vi "Main FPGA 5-axis Servo 3.vi"() -> ()   [LabVIEW 2014]
uses:
  <vilib>/Motion/MotorControl/_s/nism.encoder.config.ctl
  <vilib>/Motion/MotorControl/_s/nism.encoder.incremental.config.ctl
  <vilib>/Motion/MotorControl/_s/nism.incremental.indexCriteria.ctl
  <vilib>/Motion/MotorControl/_s/nism.mdoMemoryOffsets.ctl
  <vilib>/Motion/MotorControl/_s/nism.pid.gains.fxp.18.ctl
  <vilib>/Motion/MotorControl/_s/nism.pi.v.outputRange.fxp.6.12.ctl
  <vilib>/Motion/MotorControl/_s/nism.interpretControlRegister.stateTransition.ctl
  <vilib>/Platform/TimedLoop/XDataNode/timing_clust.ctl
  <vilib>/Platform/TimedLoop/XDataNode/nitl_modes.ctl
  <vilib>/Platform/TimedLoop/XDataNode/wakeup.ctl
  <vilib>/Motion/MotorControl/_s/nism.digitalInputs.portA.ctl
  <vilib>/rvi/Emulation/niFpgaGetClockAttributes.vi
  <vilib>/rvi/Emulation/niFpgaSctlEmulationGetInTimedLoop.vi
  <vilib>/rvi/Emulation/niFpgaEmulationReportErrorSimple.vi
  Global FPGA 6-axis.vi
  <vilib>/Motion/MotorControl/_s/nism.interpretControlRegister.indexed.vi
  <vilib>/rvi/Emulation/niFpgaProcessEmulError.vi
  <vilib>/Motion/MotorControl/_s/nism.mdo.read.encoder.vi
  <vilib>/Motion/MotorControl/_s/nism.mdo.read.positionLoopSyncData.vi
  <vilib>/Motion/MotorControl/_s/nism.mdo.read.splineData.vi
  <vilib>/Motion/MotorControl/_s/nism.mdo.read.single.vi
  <vilib>/Motion/MotorControl/_s/nism.generateStatusRegister.indexed.vi
  <vilib>/rvi/eio/common/nirviEmuTemplateMethod_errors.vi
  <vilib>/rvi/Emulation/niFpgaCriticalErrorInLSC.vi
  <vilib>/Motion/MotorControl/_s/nism.splineInterpolation.fxp.3.index.vi
  <vilib>/Motion/MotorControl/_s/nism.pid.simple.fxp.index.2.vi
  <vilib>/Motion/MotorControl/_s/nism.mdo.handler.indexed.vi
  <vilib>/Motion/MotorControl/_s/nism.digitalFilter.indexed.vi
  <vilib>/Motion/MotorControl/_s/nism.interpretDIOControl.portA.multiple.vi
  <vilib>/Motion/MotorControl/_s/nism.generateDIOStatus.portA.indexed.2.vi
  <vilib>/Motion/SoftMotion/Synchronization/nism.rioScan.generateSyncScan.vi
  <vilib>/Motion/MotorControl/_s/nism.incremental.p.2.vi
  <vilib>/eio/EIONode/EIONode.xnode
  <vilib>/Platform/TimedLoop/XDataNode/XDataNode.xnode
  <vilib>/Motion/MotorControl/NI_SoftMotion_MotorControlIP.lvlib
  <vilib>/Platform/TimedLoop/XDataNode/XDNodeRunTimeDep.lvlib
  <vilib>/Motion/SoftMotion/Synchronization/NI_SoftMotion_Synchronization.lvlib
  <vilib>/rvi/Analysis/measure/butterworth/XNode/niFpgaButterworthFilter.xnode
panel:
  in  "Reset Encoder 2":bool caption="reset"
  out "Velocity Feedback":i16[](array[numeric])
  out "pos. error":i16[](array[numeric])
  out "pos. error exceeded":bool[](array[boolean])
  in  "calls per sample (vel)":u16=2000 caption="calls per sample"
  out "Axis States":T1[](array[typedef])=[enum."Invalid", enum."Invalid", enum."Invalid", enum."Invalid", enum."Invalid", enum."Invalid"]
  in  "Limit Ranges":T2[](array[typedef])=[{"output low"=0.0, "output high"=0.0}, {"output low"=0.0, "output high"=0.0}, {"output low"=0.0, "output high"=0.0}, {"output low"=0.0, "output high"=0.0}, {"output low"=0.0, "output high"=0.0}, {"output low"=0.0, "output high"=0.0}]
  in  "Gains":T3[](array[typedef])=[{"kp"=0.0, "kd"=0.0, "ki"=0.0}, {"kp"=0.0, "kd"=0.0, "ki"=0.0}, {"kp"=0.0, "kd"=0.0, "ki"=0.0}, {"kp"=0.0, "kd"=0.0, "ki"=0.0}, {"kp"=0.0, "kd"=0.0, "ki"=0.0}, {"kp"=0.0, "kd"=0.0, "ki"=0.0}]
  out "AO Check":fxp<+/-,20,5>[](array[numeric])
  in  "AO Manual":fxp<+/-,20,5>[](array[numeric])=[0.0, 0.0, 0.0, 0.0, 0.0, 0.0]
  out "Position Feedback":i32[](array[numeric])
  in  "Reset Encoder 1":bool caption="reset"
  out "corrected period":u16
  in  "AO Disabled?":bool
  out "PID loop time (ticks)":u32
  in  "AO Override?":bool
  in  "position error limit":i16=10000
  out "SE value":u32 caption="value"
  in  "Memory Type":T4=90 caption="mbox memory offsets" items=["1 / Current Loop Rate"=108, "Anti-Resonance Enable Velocity"=98, "Axis Control Mode"=88, "Axis Velocity Filter Coefficient 1"=60, "Axis Velocity Filter Coefficient 2"=61, "Axis Velocity Filter Coefficient 3"=62, "Axis Velocity Filter Frequency"=59, "Captured Index Position"=68, "Captured Position"=58, "Coefficient 0"=96, "Coefficient 1"=95, "Coefficient 2"=101, "Coefficient 3"=97, "Coefficient 4"=99, "Coefficient 5"=100, "Compare Mode"=81, "Compare Period"=32, "Compare Position"=55, "Config Sent"=82, "Control Register"=33, "Control Register State Transition"=57, "Current Loop I2T Constant"=38, "Current Loop I2T Current to Clamp to"=40, "Current Loop I2T Icont Limit Squared"=39, "Current Loop Integral Gain"=36, "Current Loop Proportional Gain"=35, "Current Loop Rate"=37, "Digital Input Digital Filter"=1, "Digital Output Safe State"=73, "Encoder Filter Rate (uS)"=92, "Encoder Index Active State"=65, "Encoder Index Reference Line A State"=66, "Encoder Index Reference Line B State"=67, "Encoder Line A Active State"=63, "Encoder Line B Active State"=64, "Encoder Velocity"=90, "Enforce Open-Loop Position Error Limit"=71, "Fault Codes"=45, "Fault Occurred"=41, "Forward Limit Digital Filter"=24, "Gain Set 2 Current Loop Integral Gain"=106, "Gain Set 2 Current Loop Proportional Gain"=107, "Home Switch Digital Filter"=26, "Maximum Position Error Exceeded"=69, "Motor Hall Angle 1"=12, "Motor Hall Angle 2"=13, "Motor Hall Angle 3"=14, "Motor Peak Current"=16, "Motor Peak Time"=17, "Motor Phase Current Offset(A)"=83, "Motor Phase Current Offset(B)"=84, "Motor Poles"=18, "Motor Rated Phase Current"=15, "Null"=0, "PWM Periods Per Tick"=94, "Position Capture Active State"=56, "Position Capture Condition"=30, "Position Capture Digital Filter"=31, "Position Compare Action"=27, "Position Compare Active State"=54, "Position Compare Pulse Width"=29, "Position Compare Safe State"=72, "Position Compare Window"=28, "Position Loop Period"=103, "Position Loop Position Error Limit"=70, "Position Loop Proportional Gain"=9, "Reverse Limit Digital Filter"=25, "Scan Period (nsec)"=104, "Spline Period/Trajectory Period"=44, "Spline Type"=42, "Status Register"=34, "Stepper Current Reduction Delay"=20, "Stepper Current Reduction Percentage"=19, "Stepper Microstepping Rate"=21, "Stepper Minimum Pulse Width"=22, "Stepper Reduced Current"=85, "Stepper Spline Loop Period"=23, "Torque Smoothing Gain"=102, "Torque Smoothing Phase"=105, "Trajectory Period/Spline Period"=43]
  in  "Encoder filter value (us) Manual":u16=10
  out "encoder config":T5
  in  "Velocity Filter Active?":bool
  in  "Encoder Config (Manual)":T5={"active states"={"line a active high?"=FALSE, "line b active high?"=FALSE, "index active high?"=FALSE}, "index criteria"={"a"=FALSE, "b"=FALSE, "z"=FALSE}, "vel. filter coeffs."=[0, 0, 0]} caption="encoder config"
  out "Home Limits":bool[](array[boolean])
  out "Fwd Limits":bool[](array[boolean])
  out "Rev Limits":bool[](array[boolean])
  out "Drive Enable":bool[](array[boolean])
  in  "Enable Watchdog":bool
  in  "Pet Watchdog":bool
  in  "Watchdog Timeout Period (ticks)":u64=40000000 format="%.0p"
  out "Watchdog Timed Out?":bool
  out "Time Since Last Pet":u64
  in  "Enable value":bool
  in  "Drive Enable override?":bool
  in  "Sync Value":bool
  in  "Sync Enable override?":bool
  in  "Invert direction?":bool
  out "Sync is Fault":bool
  out "Sync is Locked":bool
  # "Synchronization Loop"
  # "Control Status Loop"
  # "Notes: \n1. This VI provides the communication interface between the NI SoftMotion Engine and the LabVIEW FPGA Module. You must compile this VI for a specific FPGA target before use. After compiling, run the VI before running any of the Express VI examples. For information on moving this example to another FPGA target, refer to ni.com/info and enter info code fpgaex.\n\n2. Only use the Reset Axis button if you are unable to communicate with the axis by any other means. This button resets the device state machine and other VIs to a known state. After resetting the axis, switch the NI Scan Engine from Active Mode to Configuration Mode, then back to Active Mode, before attempting to enable the axis."
  # "(These two buttons \nare for testing\npurposes.)"
  # "(These two buttons \nare for testing\npurposes.)"
  # "Position/PID Loop"
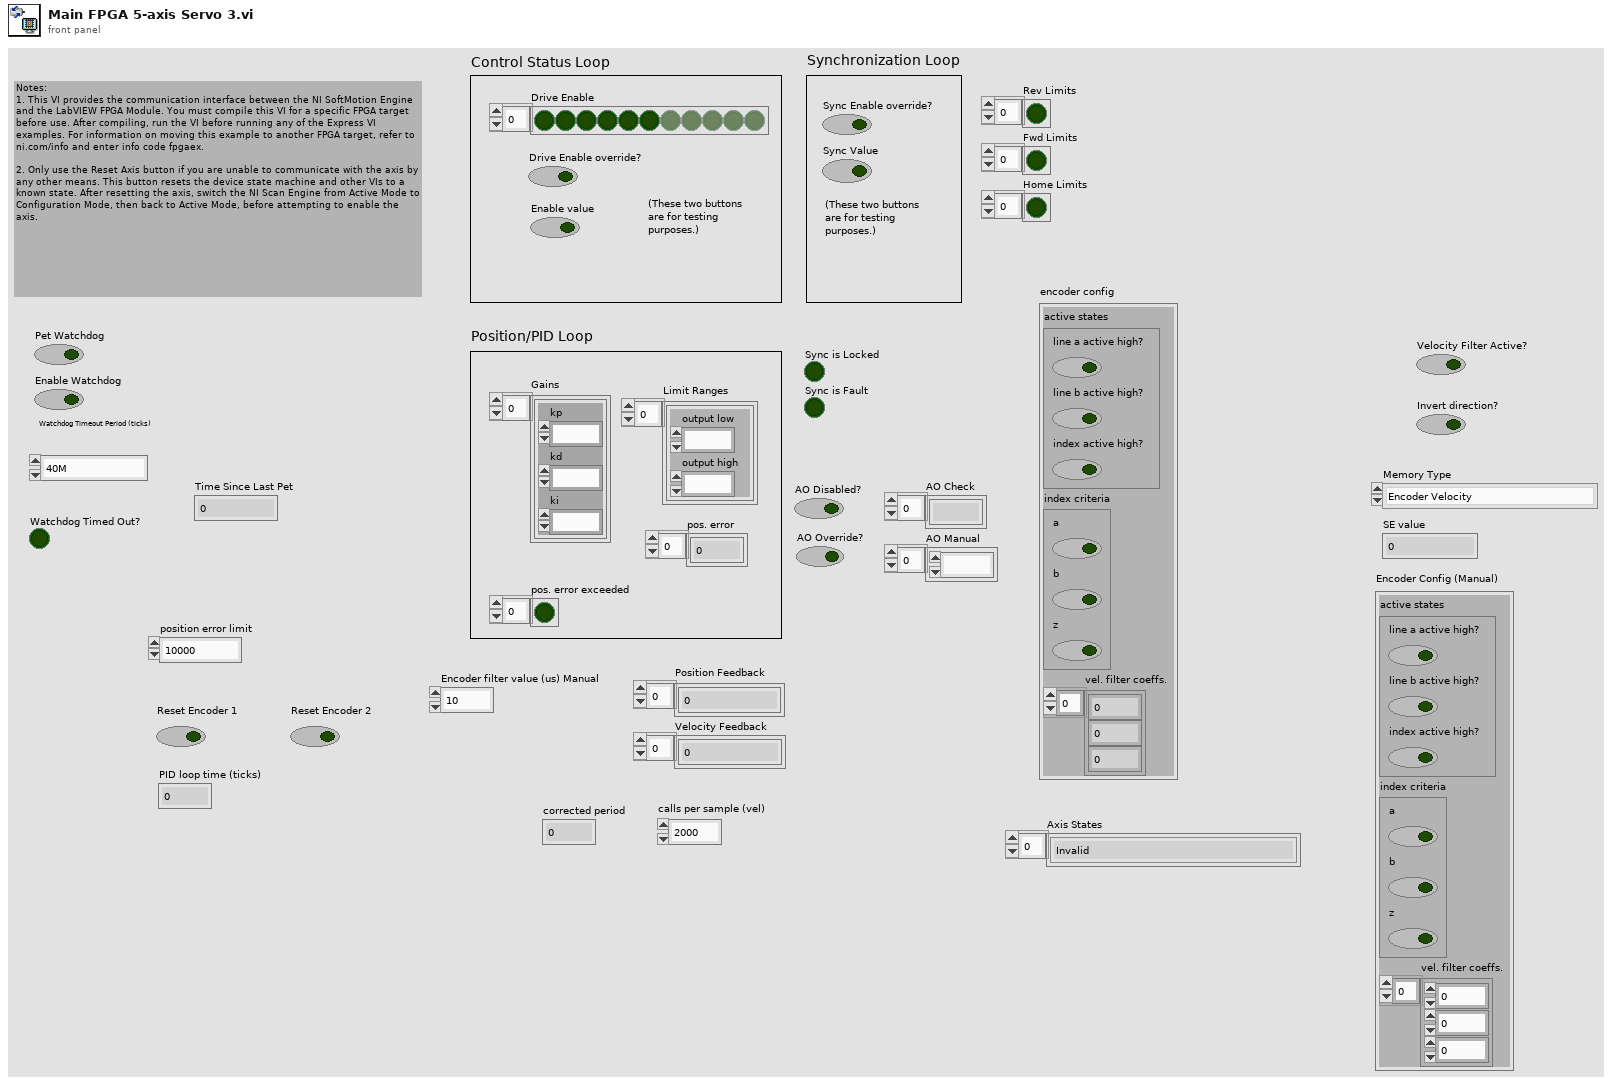
[diagram p1: front panel]
types:
  T1 = typedef "NI_SoftMotion_MotorControlIP.lvlib/nism.interpretControlRegister.stateTransition.ctl" = enum8{"Invalid", "Start --> Initializing", "Initializing --> Disabled", "Disabled --> Ready To Switch On", "Ready To Switch On --> Switched On", "Ready To Switch On --> Disable", "Switched On --> Operation Enable", "Switched On --> Ready To Switch On", "Switched On --> Disabled", "Operation Enable --> Switched On", "Operation Enable --> Ready To Switch On", "Operation Enable --> Disabled", "Fault --> Disabled", "Any --> Fault", "None"}
  T2 = typedef "NI_SoftMotion_MotorControlIP.lvlib/nism.pi.v.outputRange.fxp.6.12.ctl" = cluster{"output low":fxp<+/-,18,6>, "output high":fxp<+/-,18,6>}
  T3 = typedef "NI_SoftMotion_MotorControlIP.lvlib/nism.pid.gains.fxp.18.ctl" = cluster{"kp":fxp<+,18,7>, "kd":fxp<+,18,7>, "ki":fxp<+,18,0>}
  T4 = typedef "NI_SoftMotion_MotorControlIP.lvlib/nism.mdoMemoryOffsets.ctl" = u16
  T5 = typedef "NI_SoftMotion_MotorControlIP.lvlib/nism.encoder.config.ctl" = cluster{"active states":T6, "index criteria":T7, "vel. filter coeffs.":i32[]}
  T6 = typedef "NI_SoftMotion_MotorControlIP.lvlib/nism.encoder.incremental.config.ctl" = cluster{"line a active high?":bool, "line b active high?":bool, "index active high?":bool}
  T7 = typedef "NI_SoftMotion_MotorControlIP.lvlib/nism.incremental.indexCriteria.ctl" = cluster{"a":bool, "b":bool, "z":bool}
  T8 = typedef "XDNodeRunTimeDep.lvlib/timing_clust.ctl" = cluster{"Expected End [f-1]":u64, "Actual End [f-1]":u64, "Finished Late? [f-1]":bool, "Expected End [i-1]":u64, "Actual End [i-1]":u64, "Finished Late? [i-1]":bool, "Expected Start [i]":u64, "Actual Start [i]":u64, "Expected Start [f]":u64, "Actual Start [f]":u64, "Source Name":string, "Structure Name":string, "Period":i64, "Deadline":i64, "Offset":i64, "Start":i64, "Priority":i32, "Timeout":i32, "Mode":T9, "Wakeup Reason":T10, "Error":errorcluster, "Source Type":string, "Secondary Source Type":string, "Global End Time":u64, "Global Start Time":u64, "Frame Duration":u64, "Iteration Duration":u64, "Assigned CPU":i32, "I/O Scan Engine Mode":u32}
  T9 = typedef "XDNodeRunTimeDep.lvlib/nitl_modes.ctl" = enum32{"No Change", "Process missed periods, maintain original phase", "Discard missed periods, maintain original phase", "Process missed periods, ignore original phase", "Discard missed periods, ignore original phase"}
  T10 = typedef "XDNodeRunTimeDep.lvlib/wakeup.ctl" = enum32{"Normal", "Aborted", "Asynchronous wakeup", "Timing source error", "Timed loop error", "Timeout"}
  T11 = typedef "NI_SoftMotion_MotorControlIP.lvlib/nism.digitalInputs.portA.ctl" = cluster{"reverse limit":bool, "forward limit":bool, "home switch":bool, "digital input 0":bool, "digital input 1":bool, "digital input 2":bool, "digital input 3":bool}
  T12 = typedef "NI_SoftMotion_MotorControlIP.lvlib/nism.dio.portA.config.2.ctl" = cluster{"digital filter (us)":u16[], "safe state":T13[]}
  T13 = typedef "nism.safeStates.ctl" = enum8{"Low", "High", "No Change"}
  T14 = typedef "NI_SoftMotion_Synchronization.lvlib/nism.softmotionScan.timerConfig.ctl" = cluster{"target period (clocks)":u16, "host period / target period":u16}
  T15 = typedef "NI_SoftMotion_Synchronization.lvlib/nism.softmotionScan.timerControl.ctl" = cluster{"sm scan":bool, "sm scan count":u32, "sm scan enabled":bool}
  T16 = typedef "NI_SoftMotion_MotorControlIP.lvlib/nism.mdo.splineData.ctl" = cluster{"spline type":T17, "traj per/spline per":u16, "spline per/traj per":fxp<+,32,0>}
  T17 = typedef "NI_SoftMotion_MotorControlIP.lvlib/nism.splineInterpolation.type.ctl" = u16
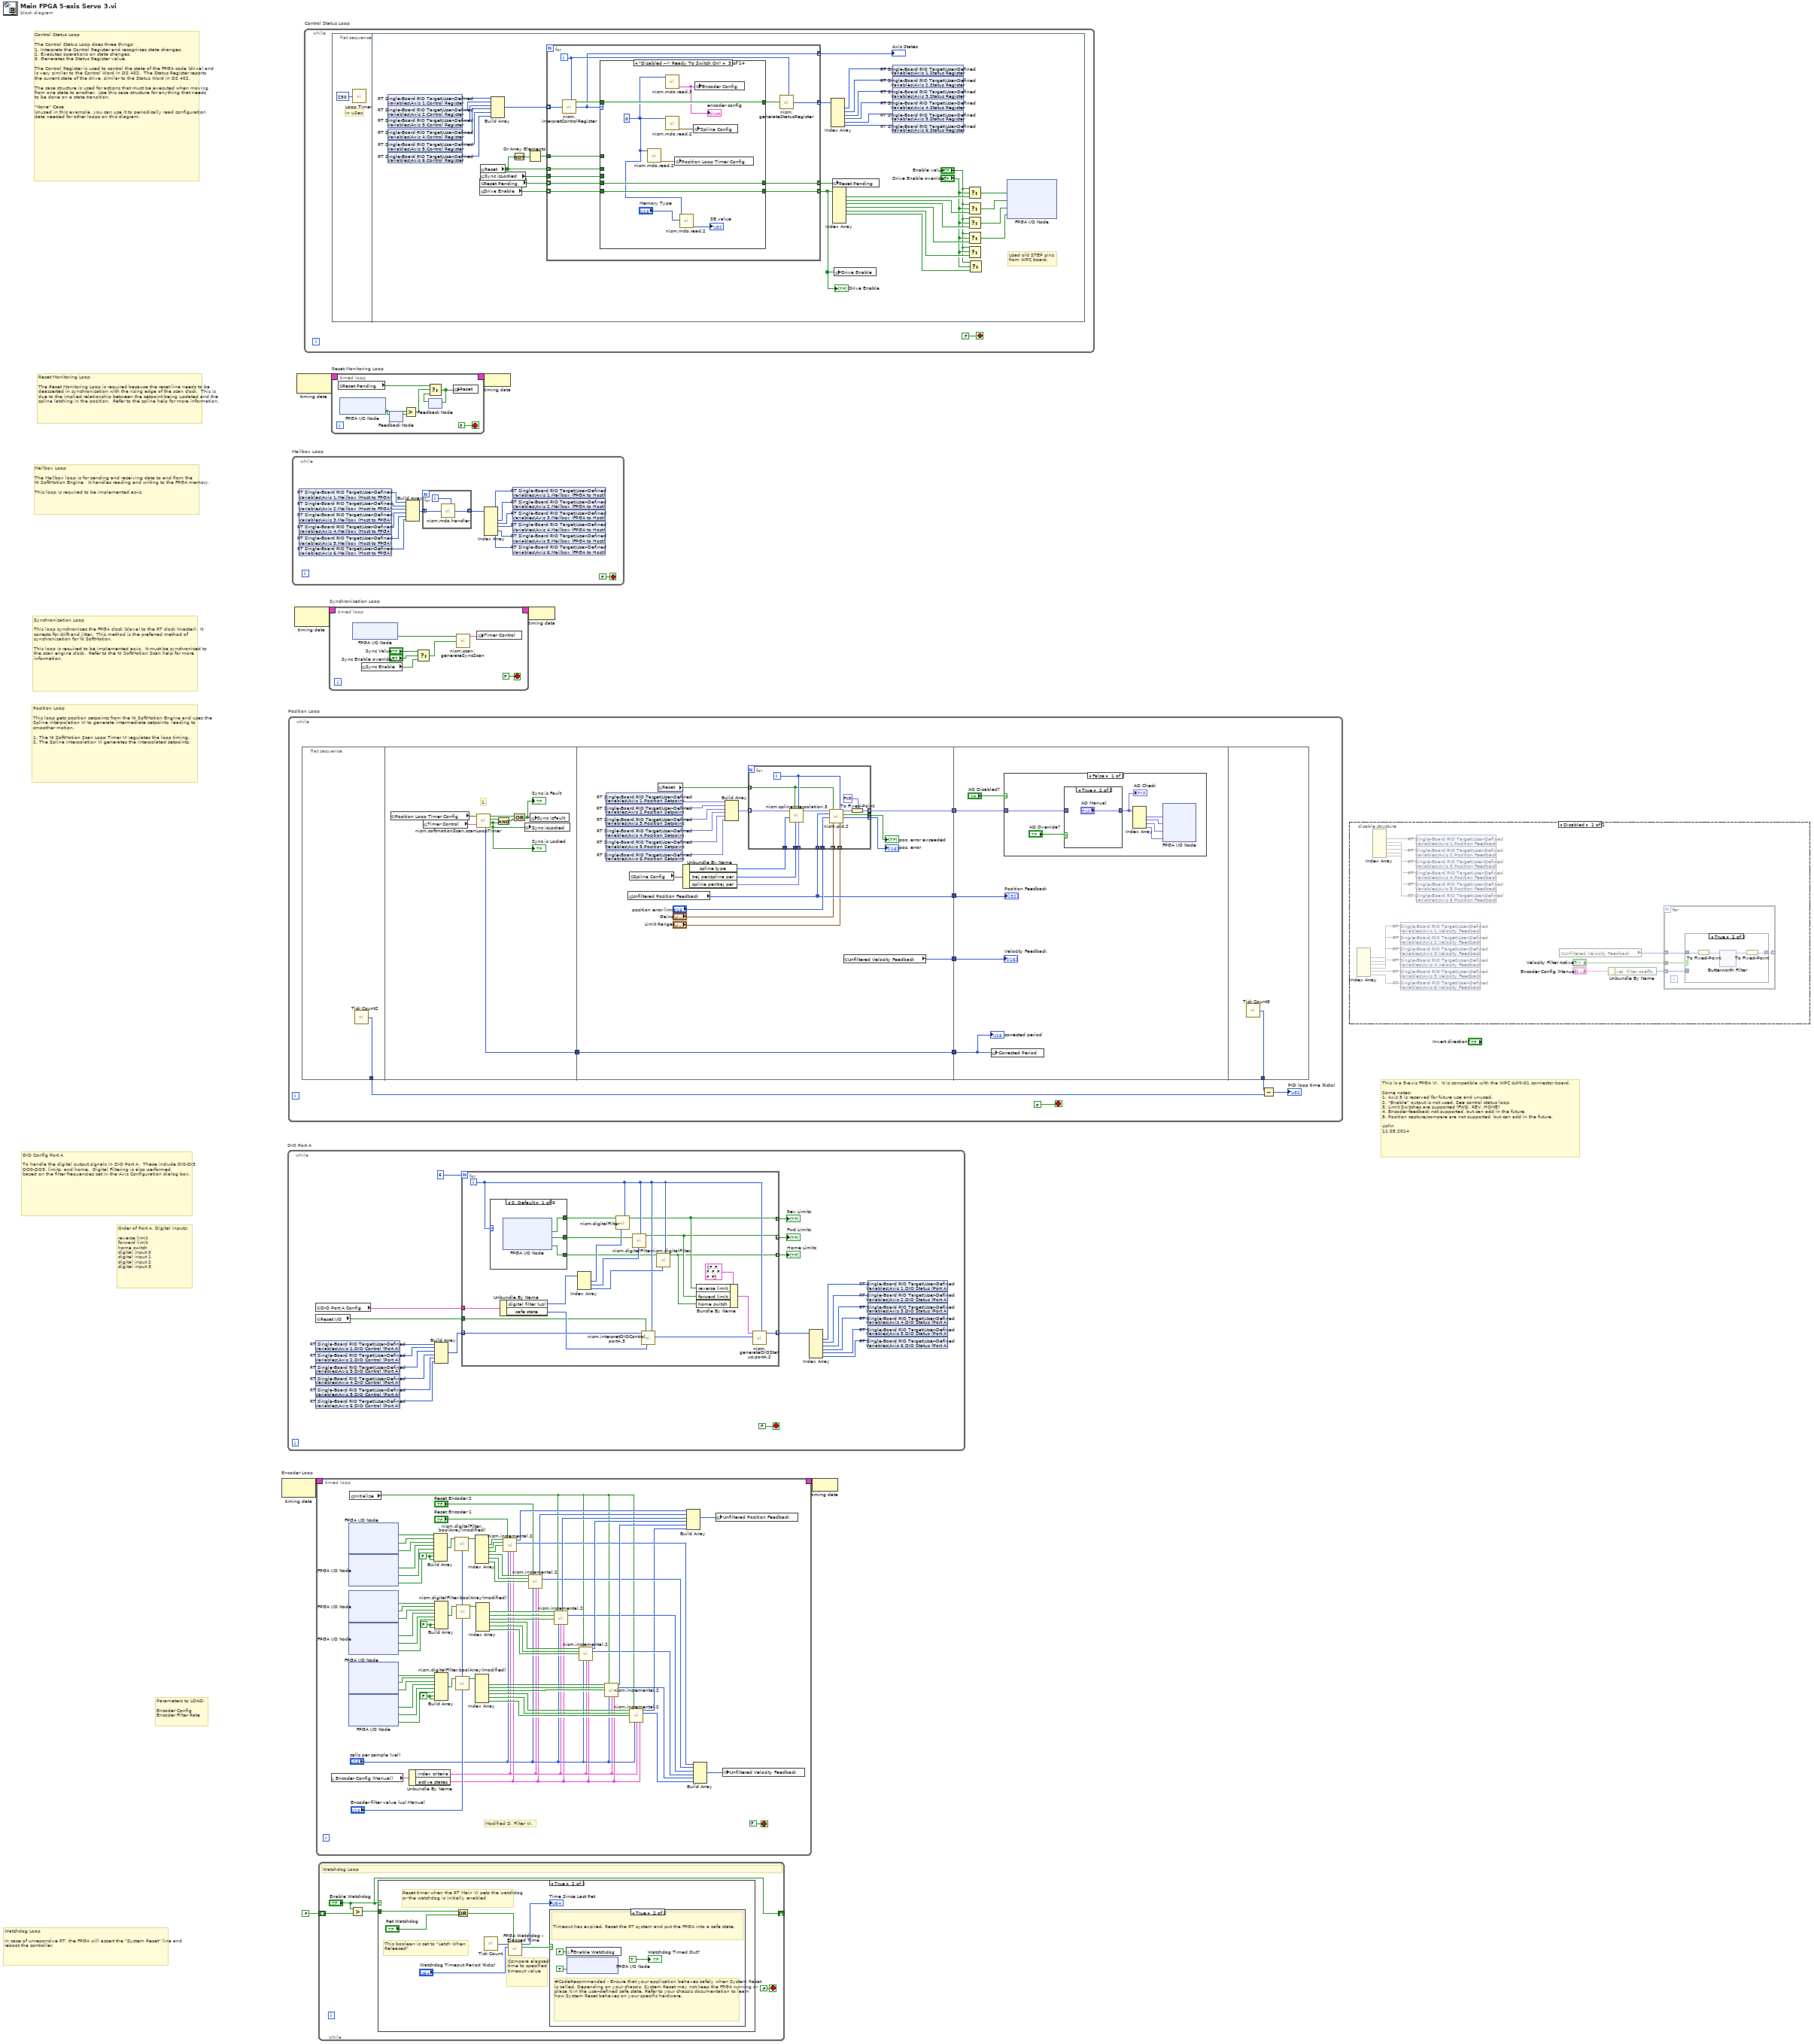
[diagram p0: block diagram]
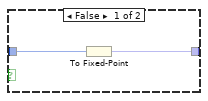
[diagram p2: hidden frame]
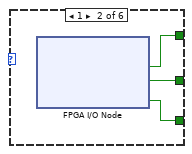
[diagram p4: hidden frame]
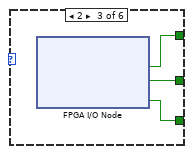
[diagram p5: hidden frame]
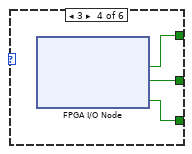
[diagram p6: hidden frame]
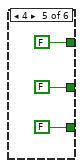
[diagram p7: hidden frame]
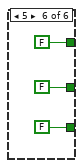
[diagram p8: hidden frame]
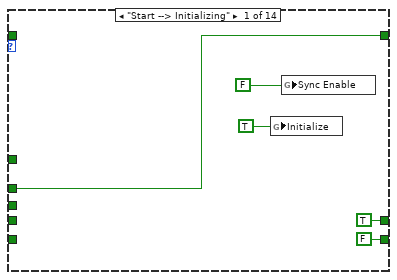
[diagram p13: hidden frame]
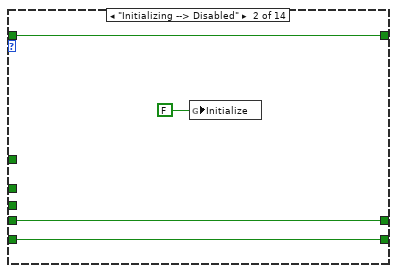
[diagram p14: hidden frame]
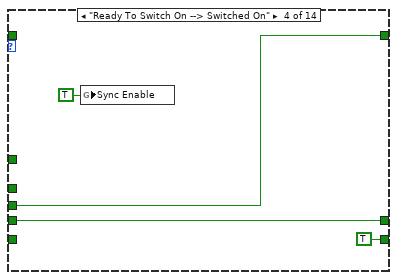
[diagram p15: hidden frame]
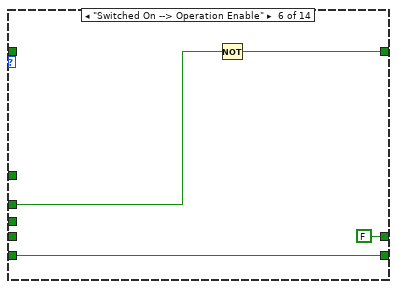
[diagram p17: hidden frame]
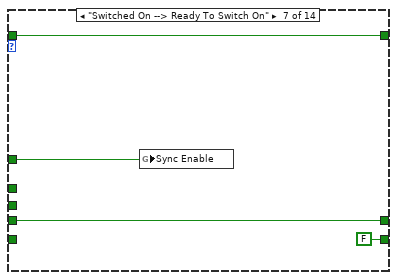
[diagram p18: hidden frame]
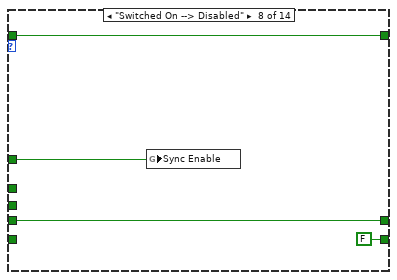
[diagram p19: hidden frame]
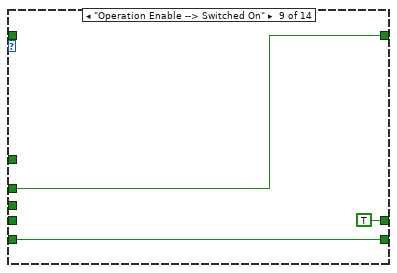
[diagram p20: hidden frame]
diagram:
  # "Parameters to LOAD:\n\nEncoder Config\nEncoder Filter Rate"
  # "This is a 5-axis FPGA VI.  It is compatible with the WPC cUMI-01 connector board.\n\nSome notes:\n1. Axis 5 is reserved for future use and unused.\n2. \"Enable\" output is not used. See control status loop.\n3. Limit Switches are supported (FWD, REV, HOME)\n4. Encoder feedback not supported, but can add in the future.\n5. Position capture/compare are not supported, but can add in the future.\n\n-John\n11.05.2014"
  # "DIO Config Port A\n\nTo handle the digital output signals in DIO Port A.  These include DI0-DI3, DO0-DO3, limits, and home.  Digital Filtering is also performed\nbased on the filter frequencies set in the Axis Configuration dialog box."
  # "Order of Port A, Digital Inputs:\n\nreverse limit\nforward limit\nhome switch\ndigital input 0\ndigital input 1\ndigital input 2\ndigital input 3"
  # "Watchdog Loop\n\nIn case of unreponsive RT, the FPGA will assert the \"System Reset\" line and reboot the controller."
  # "Position Loop\n\nThis loop gets position setpoints from the NI SoftMotion Engine and uses the Spline Interpolation VI to generate intermediate setpoints, leading to smoother motion.\n\n1. The NI SoftMotion Scan Loop Timer VI regulates the loop timing. \n2. The Spline Interpolation VI generates the interpolated setpoints."
  # "Synchronization Loop\n\nThis loop synchronizes the FPGA clock (slave) to the RT clock (master).  It corrects for drift and jitter.  This method is the preferred method of synchronization for NI SoftMotion.\n\nThis loop is required to be implemented as-is.  It must be synchronized to the scan engine clock.  Refer to the NI SoftMotion Scan help for more information."
  # "Mailbox Loop\n\nThe Mailbox loop is for sending and receiving data to and from the \nNI SoftMotion Engine.  It handles reading and writing to the FPGA memory.\n\nThis loop is required to be implemented as-is."
  # "Reset Monitoring Loop\n\nThe Reset Monitoring Loop is required because the reset line needs to be deasserted in synchronization with the rising edge of the scan clock.  This is due to the implied relationship between the setpoint being updated and the spline latching in the position.  Refer to the spline help for more information."
  # "Control Status Loop\n\nThe Control Status Loop does three things:\n1. Interprets the Control Register and recognizes state changes.\n2. Executes operations on state changes.\n3. Generates the Status Register value.\n\nThe Control Register is used to control the state of the FPGA code (drive) and is very similar to the Control Word in DS 402.  The Status Register reports the current state of the drive, similar to the Status Word in DS 402.\n\nThe case structure is used for actions that must be executed when moving from one state to another.  Use this case structure for anything that needs to be done on a state transition.\n\n\"None\" Case\nUnused in this example, you can use it to periodically read configuration data needed for other loops on this diagram."
  n1 = node-c288() -> (w2:T8)  [unwired: 1 in]
  n2 = while "DIO Port A" {
    stop <- FALSE stop-if-true
    n3 = global read "Global FPGA 6-axis.vi" "DIO Port A Config"() -> (w27:T12)
    n4 = global read "Global FPGA 6-axis.vi" "Reset I/O"() -> (w26:bool)
    n5 = shared-variable "RT Single-Board RIO Target\\User-Defined Variables\\Axis 1.DIO Control (Port A)"() -> (w24:u32)  [unwired: 1 in, 1 out]
    n6 = shared-variable "RT Single-Board RIO Target\\User-Defined Variables\\Axis 2.DIO Control (Port A)"() -> (w23:u32)  [unwired: 1 in, 1 out]
    n7 = shared-variable "RT Single-Board RIO Target\\User-Defined Variables\\Axis 3.DIO Control (Port A)"() -> (w22:u32)  [unwired: 1 in, 1 out]
    n8 = shared-variable "RT Single-Board RIO Target\\User-Defined Variables\\Axis 4.DIO Control (Port A)"() -> (w21:u32)  [unwired: 1 in, 1 out]
    n9 = shared-variable "RT Single-Board RIO Target\\User-Defined Variables\\Axis 5.DIO Control (Port A)"() -> (w20:u32)  [unwired: 1 in, 1 out]
    n10 = shared-variable "RT Single-Board RIO Target\\User-Defined Variables\\Axis 6.DIO Control (Port A)"() -> (w9:u32)  [unwired: 1 in, 1 out]
    n11 = Build Array(w24, w23, w22, w21, w20, w9) -> (w19:u32[])
    n12 = for {
      N: 6 -> [_]
      tunnel: [w46] -> w13 mode=indexing
      tunnel: w19 -> [w45] mode=indexing
      tunnel: w27 -> [w42]
      tunnel: w26 -> [w40]
      tunnel: [w31] -> w12 mode=indexing
      tunnel: [w30] -> w11 mode=indexing
      tunnel: [w29] -> w10 mode=indexing
      i -> [w35]
      n13 = case shown="0, Default" w35 {
        tunnel: [w50 w53 w56 w59 FALSE ("RMC/DIO44") FALSE ("RMC/DIO44")] -> w34
        tunnel: [w48 w51 w54 w57 FALSE ("RMC/DIO61") FALSE ("RMC/DIO61")] -> w33
        tunnel: [w49 w52 w55 w58 FALSE ("RMC/DIO77") FALSE ("RMC/DIO77")] -> w32
        frame 0, Default {
          n14 = xnode "FPGA I/O Node"() -> ("RMC/DIO29"=w50:bool, "RMC/DIO93"=w49:bool, "RMC/DIO11"=w48:bool)  [unwired: 3 in, 3 out]
        }
        frame 1 {
          n15 = xnode "FPGA I/O Node"() -> ("RMC/DIO44"=w53:bool, "RMC/DIO77"=w52:bool, "RMC/DIO61"=w51:bool)  [unwired: 3 in, 3 out]
        }
        frame 2 {
          n16 = xnode "FPGA I/O Node"() -> ("RMC/DIO31"=w56:bool, "RMC/DIO95"=w55:bool, "RMC/DIO13"=w54:bool)  [unwired: 3 in, 3 out]
        }
        frame 3 {
          n17 = xnode "FPGA I/O Node"() -> ("RMC/DIO47"=w59:bool, "RMC/DIO46"=w58:bool, "RMC/DIO79"=w57:bool)  [unwired: 3 in, 3 out]
        }
        frame 4 {
        }
        frame 5 {
        }
      }
      n18 = Unbundle By Name(w42) -> ("digital filter (us)"=w36:u16[], "safe state"=w41:T13[])
      n19 = Index Array(array=w36) -> (element #1=w37:u16, element #2=w38:u16, element #3=w39:u16)  [unwired: 3 in]
      n20 = call-poly <vilib>:"nism.digitalFilter.vi"("index"=w35, "filter value (us)"=w37, "input signal"=w34) -> ("output signal"=w31:bool)  [unwired: 8 in]
      n21 = call-poly <vilib>:"nism.digitalFilter.vi"("index"=w35, "filter value (us)"=w38, "input signal"=w32) -> ("output signal"=w30:bool)  [unwired: 8 in]
      n22 = call-poly <vilib>:"nism.interpretDIOControl.portA.3.vi"("index"=w35, "safe state"=w41, "reset"=w40, "dio control(port a)"=w45) -> ("reset latches"=w47:u8)  [unwired: 6 in, 1 out]
      n23 = call-poly <vilib>:"nism.digitalFilter.vi"("index"=w35, "filter value (us)"=w39, "input signal"=w33) -> ("output signal"=w29:bool)  [unwired: 8 in]
      n24 = Bundle By Name(cluster=T11 {"reverse limit"=FALSE, "forward limit"=FALSE, "home switch"=FALSE, "digital input 0"=FALSE, "digital input 1"=FALSE, "digital input 2"=FALSE, "digital input 3"=FALSE} ("$(driveInterface.digitalInputs.shortName)"), "reverse limit"=w31, "forward limit"=w30, "home switch"=w29) -> (w43:T11)
      n25 = call-poly <vilib>:"nism.generateDIOStatus.portA.2.vi"("index"=w35, "reset latches"=w47, "digital inputs"=w43) -> ("dio status(port a)"=w46:u32)  [unwired: 8 in]
    }
    "Rev Limits" <- w12
    "Fwd Limits" <- w11
    "Home Limits" <- w10
    n26 = Index Array(array=w13) -> (element #1=w18:u32, element #2=w17:u32, element #3=w16:u32, element #4=w15:u32, element #5=w14:u32, element #6=w8:u32)  [unwired: 6 in]
    n27 = shared-variable "RT Single-Board RIO Target\\User-Defined Variables\\Axis 1.DIO Status (Port A)"(w18) -> ()  [unwired: 1 in, 1 out]
    n28 = shared-variable "RT Single-Board RIO Target\\User-Defined Variables\\Axis 2.DIO Status (Port A)"(w17) -> ()  [unwired: 1 in, 1 out]
    n29 = shared-variable "RT Single-Board RIO Target\\User-Defined Variables\\Axis 3.DIO Status (Port A)"(w16) -> ()  [unwired: 1 in, 1 out]
    n30 = shared-variable "RT Single-Board RIO Target\\User-Defined Variables\\Axis 4.DIO Status (Port A)"(w15) -> ()  [unwired: 1 in, 1 out]
    n31 = shared-variable "RT Single-Board RIO Target\\User-Defined Variables\\Axis 5.DIO Status (Port A)"(w14) -> ()  [unwired: 1 in, 1 out]
    n32 = shared-variable "RT Single-Board RIO Target\\User-Defined Variables\\Axis 6.DIO Status (Port A)"(w8) -> ()  [unwired: 1 in, 1 out]
  }
  n33 = while "Position Loop" {
    stop <- FALSE stop-if-true
    n34 = flat-sequence {
      tunnel: [w75] -> w69
      tunnel: [w76] -> w72
      tunnel: [w100] -> w73
      tunnel: w72 -> [w100]
      tunnel: [w90] -> w71
      tunnel: [w94] -> w67
      tunnel: [w84] -> w66
      tunnel: w73 -> [w125]
      tunnel: w71 -> [w122]
      tunnel: w67 -> [w124]
      tunnel: w66 -> [w121]
      tunnel: [w135] -> w70
      frame #0 {
        n35 = call "Tick Count2"() -> ("Tick Count(Ticks)"=w75:u32)
      }
      frame #1 {
        # "1."
        n36 = global read "Global FPGA 6-axis.vi" "Position Loop Timer Config"() -> (w78:T14)
        n37 = global read "Global FPGA 6-axis.vi" "Timer Control"() -> (w77:T15)
        n38 = call <vilib>:"nism.softmotionScan.scanLoopTimer.vi"("timer control"=w77, "timer config"=w78) -> ("scan running?"=w80:bool, "finished late?"=w82:bool, "fault occurred?"=w83:bool, "corrected period"=w76:u16)  [unwired: 5 in, 1 out]
        "Sync is Locked" <- w80
        n39 = Compound Arithmetic op=AND(w82, w80) -> (w81:bool)
        n40 = Compound Arithmetic op=OR(w83, w81) -> (w79:bool)
        "Sync is Fault" <- w79
        n41 = global write "Global FPGA 6-axis.vi" "Sync isLocked"(w80) -> ()
        n42 = global write "Global FPGA 6-axis.vi" "Sync isFault"(w79) -> ()
      }
      frame #2 {
        n43 = shared-variable "RT Single-Board RIO Target\\User-Defined Variables\\Axis 1.Position Setpoint"() -> (w95:fxp<+/-,64,32>)  [unwired: 1 in, 1 out]
        n44 = shared-variable "RT Single-Board RIO Target\\User-Defined Variables\\Axis 2.Position Setpoint"() -> (w99:fxp<+/-,64,32>)  [unwired: 1 in, 1 out]
        n45 = shared-variable "RT Single-Board RIO Target\\User-Defined Variables\\Axis 3.Position Setpoint"() -> (w98:fxp<+/-,64,32>)  [unwired: 1 in, 1 out]
        n46 = shared-variable "RT Single-Board RIO Target\\User-Defined Variables\\Axis 4.Position Setpoint"() -> (w97:fxp<+/-,64,32>)  [unwired: 1 in, 1 out]
        n47 = shared-variable "RT Single-Board RIO Target\\User-Defined Variables\\Axis 5.Position Setpoint"() -> (w96:fxp<+/-,64,32>)  [unwired: 1 in, 1 out]
        n48 = shared-variable "RT Single-Board RIO Target\\User-Defined Variables\\Axis 6.Position Setpoint"() -> (w87:fxp<+/-,64,32>)  [unwired: 1 in, 1 out]
        n49 = global read "Global FPGA 6-axis.vi" "Unfiltered Position Feedback"() -> (w90:i32[])
        n50 = global read "Global FPGA 6-axis.vi" "Spline Config"() -> (w101:T16)
        n51 = global read "Global FPGA 6-axis.vi" "Reset"() -> (w92:bool[])
        n52 = Unbundle By Name(w101) -> ("spline type"=w104:T17, "traj per/spline per"=w103:u16, "spline per/traj per"=w102:fxp<+,32,0>)
        n53 = Build Array(w95, w99, w98, w97, w96, w87) -> (w93:fxp<+/-,64,32>[])
        n54 = for {
          tunnel: w104 -> [w120]
          tunnel: w103 -> [w119]
          tunnel: w102 -> [w118]
          tunnel: "Limit Ranges" -> [w116] mode=indexing
          tunnel: [w106] -> w94 mode=indexing
          tunnel: w93 -> [w115] mode=indexing
          tunnel: w92 -> [w113] mode=indexing
          tunnel: w90 -> [w112] mode=indexing
          tunnel: "position error limit" -> [w111]
          tunnel: [w110] -> w86 mode=indexing
          tunnel: [w109] -> w85 mode=indexing
          tunnel: "Gains" -> [w105] mode=indexing
          i -> [w114]
          n55 = call-poly <vilib>:"nism.splineInterpolation.3.vi"("1 / calls per sample"=w118, "index"=w114, "calls per sample"=w119, "reset"=w113, "spline type"=w120, "x"=w115) -> ("xi"=w117:fxp<+/-,64,32>)  [unwired: 4 in, 1 out]
          n56 = call-poly <vilib>:"nism.pid.2.vi"("position setpoint"=w117, "position feedback"=w112, "position error limit"=w111, "reset"=w113, "gains"=w105, "index"=w114, "output range"=w116) -> ("current setpoint"=w107:fxp<+/-,18,6>, "pos. error exceeded"=w110:bool, "position error"=w109:i16)  [unwired: 10 in]
          n57 = To Fixed-Point(fixed-point type=fxp<+/-,20,5> 0.0 ("AO 1"), number=w107) -> (fixed-point=w106:fxp<+/-,20,5>)
        }
        "pos. error exceeded" <- w86
        "pos. error" <- w85
        n58 = global read "Global FPGA 6-axis.vi" "Unfiltered Velocity Feedback"() -> (w84:i16[])
      }
      frame #3 {
        n59 = global write "Global FPGA 6-axis.vi" "Corrected Period"(w125) -> ()
        n60 = case shown="False" "AO Disabled?" {
          tunnel: w124 -> [w131 _]
          frame False {
            n61 = case shown="True" "AO Override?" {
              tunnel: w131 -> [w133 _]
              tunnel: [w133 "AO Manual"] -> w130
              frame False {
              }
              frame True {
              }
            }
            "AO Check" <- w130
            n62 = Index Array(array=w130) -> (element #1=w129:fxp<+/-,20,5>, element #2=w128:fxp<+/-,20,5>, element #3=w127:fxp<+/-,20,5>, element #4=w126:fxp<+/-,20,5>)  [unwired: 4 in]
            n63 = xnode "FPGA I/O Node"("AO0"=w129, "AO1"=w128, "AO2"=w127, "AO3"=w126) -> ()  [unwired: 4 in, 4 out]
          }
          frame True {
          }
        }
        "corrected period" <- w125
        "Position Feedback" <- w122
        "Velocity Feedback" <- w121
      }
      frame #4 {
        n64 = call "Tick Count3"() -> ("Tick Count(Ticks)"=w135:u32)
      }
    }
    n65 = Subtract(x=w70, y=w69) -> (x-y=→"PID loop time (ticks)":u32)
  }
  n66 = while "Mailbox Loop" {
    stop <- FALSE stop-if-true
    n67 = shared-variable "RT Single-Board RIO Target\\User-Defined Variables\\Axis 1.Mailbox (Host to FPGA)"() -> (w147:u64)  [unwired: 1 in, 1 out]
    n68 = shared-variable "RT Single-Board RIO Target\\User-Defined Variables\\Axis 2.Mailbox (Host to FPGA)"() -> (w146:u64)  [unwired: 1 in, 1 out]
    n69 = shared-variable "RT Single-Board RIO Target\\User-Defined Variables\\Axis 3.Mailbox (Host to FPGA)"() -> (w145:u64)  [unwired: 1 in, 1 out]
    n70 = shared-variable "RT Single-Board RIO Target\\User-Defined Variables\\Axis 4.Mailbox (Host to FPGA)"() -> (w144:u64)  [unwired: 1 in, 1 out]
    n71 = shared-variable "RT Single-Board RIO Target\\User-Defined Variables\\Axis 5.Mailbox (Host to FPGA)"() -> (w143:u64)  [unwired: 1 in, 1 out]
    n72 = shared-variable "RT Single-Board RIO Target\\User-Defined Variables\\Axis 6.Mailbox (Host to FPGA)"() -> (w136:u64)  [unwired: 1 in, 1 out]
    n73 = Build Array(w147, w146, w145, w144, w143, w136) -> (w149:u64[])
    n74 = for {
      tunnel: w149 -> [w153] mode=indexing
      tunnel: [w152] -> w148 mode=indexing
      i -> [w151]
      n75 = call-poly <vilib>:"nism.mdo.handler.vi"("mbox (host to fpga)"=w153, "axis index"=w151) -> ("mbox (fpga to host)"=w152:u64)  [unwired: 7 in]
    }
    n76 = Index Array(array=w148) -> (element #1=w142:u64, element #2=w141:u64, element #3=w140:u64, element #4=w139:u64, element #5=w138:u64, element #6=w137:u64)  [unwired: 6 in]
    n77 = shared-variable "RT Single-Board RIO Target\\User-Defined Variables\\Axis 1.Mailbox (FPGA to Host)"(w142) -> ()  [unwired: 1 in, 1 out]
    n78 = shared-variable "RT Single-Board RIO Target\\User-Defined Variables\\Axis 2.Mailbox (FPGA to Host)"(w141) -> ()  [unwired: 1 in, 1 out]
    n79 = shared-variable "RT Single-Board RIO Target\\User-Defined Variables\\Axis 3.Mailbox (FPGA to Host)"(w140) -> ()  [unwired: 1 in, 1 out]
    n80 = shared-variable "RT Single-Board RIO Target\\User-Defined Variables\\Axis 4.Mailbox (FPGA to Host)"(w139) -> ()  [unwired: 1 in, 1 out]
    n81 = shared-variable "RT Single-Board RIO Target\\User-Defined Variables\\Axis 5.Mailbox (FPGA to Host)"(w138) -> ()  [unwired: 1 in, 1 out]
    n82 = shared-variable "RT Single-Board RIO Target\\User-Defined Variables\\Axis 6.Mailbox (FPGA to Host)"(w137) -> ()  [unwired: 1 in, 1 out]
  }
  n83 = node-c288() -> (w7:T8)  [unwired: 1 in]
  n84 = node-c288() -> (w5:T8)  [unwired: 1 in]
  n85 = while "Control Status Loop" {
    stop <- FALSE stop-if-true
    n86 = flat-sequence {
      frame #0 {
        # "in uSec"
        n87 = call "Loop Timer"("Count(uSec)"=u32 250) -> ()  [unwired: 1 out]
      }
      frame #1 {
        # "Used old STEP pins\nfrom WPC board."
        n88 = shared-variable "RT Single-Board RIO Target\\User-Defined Variables\\Axis 1.Control Register"() -> (w180:u32)  [unwired: 1 in, 1 out]
        n89 = shared-variable "RT Single-Board RIO Target\\User-Defined Variables\\Axis 2.Control Register"() -> (w179:u32)  [unwired: 1 in, 1 out]
        n90 = shared-variable "RT Single-Board RIO Target\\User-Defined Variables\\Axis 3.Control Register"() -> (w178:u32)  [unwired: 1 in, 1 out]
        n91 = shared-variable "RT Single-Board RIO Target\\User-Defined Variables\\Axis 4.Control Register"() -> (w177:u32)  [unwired: 1 in, 1 out]
        n92 = shared-variable "RT Single-Board RIO Target\\User-Defined Variables\\Axis 5.Control Register"() -> (w176:u32)  [unwired: 1 in, 1 out]
        n93 = shared-variable "RT Single-Board RIO Target\\User-Defined Variables\\Axis 6.Control Register"() -> (w160:u32)  [unwired: 1 in, 1 out]
        n94 = global read "Global FPGA 6-axis.vi" "Reset Pending"() -> (w184:bool[])
        n95 = global read "Global FPGA 6-axis.vi" "Drive Enable"() -> (w183:bool[])
        n96 = global read "Global FPGA 6-axis.vi" "Reset"() -> (w185:bool[])
        n97 = global read "Global FPGA 6-axis.vi" "Sync isLocked"() -> (w190:bool)
        n98 = Build Array(w180, w179, w178, w177, w176, w160) -> (w189:u32[])
        n99 = Not(x=w185) -> (.not. x?=w187:bool[])
        n100 = Or Array Elements(Boolean array=w187) -> (logical OR=w186:bool)
        n101 = for {
          tunnel: w185 -> [w199] mode=indexing
          tunnel: w190 -> [w198]
          tunnel: w189 -> [w200] mode=indexing
          tunnel: [w197] -> w181 mode=indexing
          tunnel: [w196] -> w188 mode=indexing
          tunnel: [w195] -> w182 mode=indexing
          tunnel: w186 -> [w194]
          tunnel: w184 -> [w193] mode=indexing
          tunnel: w183 -> [w192] mode=indexing
          tunnel: [w191] -> w161 mode=indexing
          i -> [w201]
          n102 = call-poly <vilib>:"nism.interpretControlRegister.vi"("control register"=w200, "axis index"=w201) -> ("transition occurred"=w202:bool, "state transition"=w191:T1)  [unwired: 6 in]
          n103 = case shown="\"Disabled --> Ready To Switch On\"" w191 {
            tunnel: w202 -> [_ w212 w221 _ w228 _ w236 w240 _ _ _ _ w260 _]
            tunnel: [w208 w212 w221 w223 w228 w232 w236 w240 w242 w245 w249 w253 w259 _] -> w203
            tunnel: w199 -> [w208 _ _ _ _ w231 _ _ w242 w245 w249 w253 _ _]
            tunnel: w198 -> [_ _ _ w223 _ _ _ _ _ _ _ _ _ _]
            tunnel: [TRUE ("Write.Reset Pending") w211 w218 w222 w227 FALSE ("Write.Reset Pending") w233 w237 TRUE ("Write.Reset Pending") TRUE ("Write.Reset Pending") TRUE ("Write.Reset Pending") TRUE ("Write.Reset Pending") w257 w262] -> w196
            tunnel: [FALSE ("Write.Drive Enable") w210 w217 TRUE ("Write.Drive Enable") w226 w229 FALSE ("Write.Drive Enable") FALSE ("Write.Drive Enable") w241 FALSE ("Write.Drive Enable") FALSE ("Write.Drive Enable") FALSE ("Write.Drive Enable") w256 w261] -> w195
            tunnel: w194 -> [_ _ _ _ _ _ w234 w238 _ w244 w248 w252 w258 _]
            tunnel: w193 -> [_ w211 w218 w222 w227 _ w233 w237 _ _ _ _ w257 w262]
            tunnel: w192 -> [_ w210 w217 _ w226 w229 _ _ w241 _ _ _ w256 w261]
            frame "Start --> Initializing" {
              n104 = global write "Global FPGA 6-axis.vi" "Initialize"(TRUE ("Initialize")) -> ()
              n105 = global write "Global FPGA 6-axis.vi" "Sync Enable"(FALSE ("Sync Enable")) -> ()
            }
            frame "Initializing --> Disabled" {
              n106 = global write "Global FPGA 6-axis.vi" "Initialize"(FALSE ("Initialize")) -> ()
            }
            frame "Disabled --> Ready To Switch On" {
              w213 = 0 ("axis index")
              n107 = call-poly <vilib>:"nism.mdo.read.2.vi"("axis index"=w213) -> ("position loop sync"=w219:T14)  [unwired: 10 in]
              n108 = call-poly <vilib>:"nism.mdo.read.3.vi"("axis index"=w213) -> ("encoder config"=w216:T5)  [unwired: 10 in]
              "encoder config" <- w216
              n109 = call-poly <vilib>:"nism.mdo.read.2.vi"("axis index"=w213) -> ("spline"=w220:T16)  [unwired: 10 in]
              n110 = global write "Global FPGA 6-axis.vi" "Position Loop Timer Config"(w219) -> ()
              n111 = call-poly <vilib>:"nism.mdo.read.2.vi"("mbox memory offsets"="Memory Type", "axis index"=w213) -> ("value"=→"SE value":u32)  [unwired: 9 in]
              n112 = global write "Global FPGA 6-axis.vi" "Spline Config"(w220) -> ()
              n113 = global write "Global FPGA 6-axis.vi" "Encoder Config"(w216) -> ()
            }
            frame "Ready To Switch On --> Switched On" {
              n114 = global write "Global FPGA 6-axis.vi" "Sync Enable"(TRUE ("Sync Enable")) -> ()
            }
            frame "Ready To Switch On --> Disable" {
            }
            frame "Switched On --> Operation Enable" {
              n115 = Not(x=w231) -> (.not. x?=w232:bool)
            }
            frame "Switched On --> Ready To Switch On" {
              n116 = global write "Global FPGA 6-axis.vi" "Sync Enable"(w234) -> ()
            }
            frame "Switched On --> Disabled" {
              n117 = global write "Global FPGA 6-axis.vi" "Sync Enable"(w238) -> ()
            }
            frame "Operation Enable --> Switched On" {
            }
            frame "Operation Enable --> Ready To Switch On" {
              n118 = global write "Global FPGA 6-axis.vi" "Sync Enable"(w244) -> ()
            }
            frame "Operation Enable --> Disabled" {
              n119 = global write "Global FPGA 6-axis.vi" "Sync Enable"(w248) -> ()
            }
            frame "Any --> Fault" {
              n120 = global write "Global FPGA 6-axis.vi" "Sync Enable"(w252) -> ()
            }
            frame "Fault --> Disabled" {
              # "wait one cycle for clear faults to have taken effect"
              n121 = global write "Global FPGA 6-axis.vi" "Sync Enable"(w258) -> ()
              n122 = Not(x=w260) -> (.not. x?=w259:bool)
            }
            frame "None", Default {
            }
          }
          n123 = call-poly <vilib>:"nism.generateStatusRegister.vi"("transition success"=w203, "axis index"=w201) -> ("status register"=w197:u32)  [unwired: 7 in]
        }
        "Drive Enable" <- w182
        "Axis States" <- w161
        n124 = Index Array(array=w181) -> (element #1=w175:u32, element #2=w174:u32, element #3=w173:u32, element #4=w172:u32, element #5=w171:u32, element #6=w159:u32)  [unwired: 6 in]
        n125 = global write "Global FPGA 6-axis.vi" "Reset Pending"(w188) -> ()
        n126 = Index Array(array=w182) -> (element #1=w170:bool, element #2=w169:bool, element #3=w168:bool, element #4=w167:bool, element #5=w166:bool, element #6=w158:bool)  [unwired: 8 in, 2 out]
        n127 = global write "Global FPGA 6-axis.vi" "Drive Enable"(w182) -> ()
        n128 = shared-variable "RT Single-Board RIO Target\\User-Defined Variables\\Axis 1.Status Register"(w175) -> ()  [unwired: 1 in, 1 out]
        n129 = shared-variable "RT Single-Board RIO Target\\User-Defined Variables\\Axis 2.Status Register"(w174) -> ()  [unwired: 1 in, 1 out]
        n130 = shared-variable "RT Single-Board RIO Target\\User-Defined Variables\\Axis 3.Status Register"(w173) -> ()  [unwired: 1 in, 1 out]
        n131 = shared-variable "RT Single-Board RIO Target\\User-Defined Variables\\Axis 4.Status Register"(w172) -> ()  [unwired: 1 in, 1 out]
        n132 = shared-variable "RT Single-Board RIO Target\\User-Defined Variables\\Axis 5.Status Register"(w171) -> ()  [unwired: 1 in, 1 out]
        n133 = shared-variable "RT Single-Board RIO Target\\User-Defined Variables\\Axis 6.Status Register"(w159) -> ()  [unwired: 1 in, 1 out]
        n134 = Select(t="Enable value", s="Drive Enable override?", f=w170) -> (s? t:f=w165:bool)
        n135 = Select(t="Enable value", s="Drive Enable override?", f=w169) -> (s? t:f=w164:bool)
        n136 = Select(t="Enable value", s="Drive Enable override?", f=w168) -> (s? t:f=w163:bool)
        n137 = Select(t="Enable value", s="Drive Enable override?", f=w167) -> (s? t:f=w162:bool)
        n138 = Select(t="Enable value", s="Drive Enable override?", f=w166) -> ()  [unwired: 1 out]
        n139 = Select(t="Enable value", s="Drive Enable override?", f=w158) -> ()  [unwired: 1 out]
        n140 = xnode "FPGA I/O Node"("RMC/DIO28"=w165, "RMC/DIO12"=w164, "RMC/DIO30"=w163, "RMC/DIO14"=w162) -> ()  [unwired: 4 in, 4 out]
      }
    }
  }
  n141 = timed-loop "Encoder Loop" {
    timing: w2 -> [_]
    timing-out: [_] -> w1
    stop <- FALSE stop-if-true
    w287 = FALSE ("element")
    w288 = FALSE ("element")
    w304 = FALSE ("element")
    # "Modified D. Filter VI."
    n142 = local read "Encoder Config (Manual)"() -> (w275:T5)
    n143 = xnode "FPGA I/O Node"() -> ("RMC/DIO60"=w328:bool, "RMC/DIO42"=w329:bool, "RMC/DIO75"=w327:bool)  [unwired: 3 in, 3 out]
    n144 = xnode "FPGA I/O Node"() -> ("RMC/DIO59"=w309:bool, "RMC/DIO92"=w308:bool, "RMC/DIO10"=w307:bool)  [unwired: 3 in, 3 out]
    n145 = xnode "FPGA I/O Node"() -> ("RMC/DIO74"=w300:bool, "RMC/DIO27"=w299:bool, "RMC/DIO91"=w298:bool)  [unwired: 3 in, 3 out]
    n146 = xnode "FPGA I/O Node"() -> ("RMC/DIO9"=w297:bool, "RMC/DIO41"=w296:bool, "RMC/DIO26"=w295:bool)  [unwired: 3 in, 3 out]
    n147 = xnode "FPGA I/O Node"() -> ("RMC/DIO58"=w281:bool, "RMC/DIO40"=w282:bool, "RMC/DIO73"=w283:bool)  [unwired: 3 in, 3 out]
    n148 = xnode "FPGA I/O Node"() -> ("RMC/DIO57"=w284:bool, "RMC/DIO90"=w285:bool, "RMC/DIO8"=w286:bool)  [unwired: 3 in, 3 out]
    n149 = global read "Global FPGA 6-axis.vi" "Initialize"() -> (w269:bool)
    n150 = Unbundle By Name(w275) -> ("index criteria"=w265:T7, "active states"=w264:T6)
    n151 = Build Array(w328, w329, w327, w309, w308, w307, w304, w304) -> (w326:bool[])
    n152 = Build Array(w281, w282, w283, w284, w285, w286, w287, w287) -> (w280:bool[])
    n153 = Build Array(w300, w299, w298, w297, w296, w295, w288, w288) -> (w305:bool[])
    n154 = call "nism.digitalFilter.boolArray(modified).vi"("filter value (us)"="Encoder filter value (us) Manual", "input signal"=w326) -> ("output signal"=w325:bool[])  [unwired: 9 in]
    n155 = call "nism.digitalFilter.boolArray(modified).vi"("filter value (us)"="Encoder filter value (us) Manual", "input signal"=w280) -> ("output signal"=w279:bool[])  [unwired: 9 in]
    n156 = call "nism.digitalFilter.boolArray(modified).vi"("filter value (us)"="Encoder filter value (us) Manual", "input signal"=w305) -> ("output signal"=w306:bool[])  [unwired: 9 in]
    n157 = Index Array(array=w325) -> (element #1=w324:bool, element #2=w323:bool, element #3=w322:bool, element #4=w303:bool, element #5=w302:bool, element #6=w301:bool)  [unwired: 6 in]
    n158 = Index Array(array=w279) -> (element #1=w278:bool, element #2=w277:bool, element #3=w276:bool, element #4=w272:bool, element #5=w271:bool, element #6=w270:bool)  [unwired: 6 in]
    n159 = Index Array(array=w306) -> (element #1=w294:bool, element #2=w293:bool, element #3=w292:bool, element #4=w291:bool, element #5=w290:bool, element #6=w289:bool)  [unwired: 6 in]
    n160 = call-poly <vilib>:"nism.incremental.2.vi"("a phase"=w324, "reset"="Reset Encoder 1", "b phase"=w323, "z phase"=w322, "calls per sample"="calls per sample (vel)", "index criteria"=w265, "active states"=w264) -> ("encoder position"=w321:i32, "velocity"=w314:i16)  [unwired: 5 in, 2 out]
    n161 = call-poly <vilib>:"nism.incremental.2.vi"("a phase"=w303, "reset"="Reset Encoder 2", "b phase"=w302, "z phase"=w301, "calls per sample"="calls per sample (vel)", "index criteria"=w265, "active states"=w264) -> ("encoder position"=w320:i32, "velocity"=w313:i16)  [unwired: 5 in, 2 out]
    n162 = call-poly <vilib>:"nism.incremental.2.vi"("a phase"=w294, "reset"=w269, "b phase"=w293, "z phase"=w292, "calls per sample"="calls per sample (vel)", "index criteria"=w265, "active states"=w264) -> ("encoder position"=w319:i32, "velocity"=w312:i16)  [unwired: 5 in, 2 out]
    n163 = call-poly <vilib>:"nism.incremental.2.vi"("a phase"=w291, "reset"=w269, "b phase"=w290, "z phase"=w289, "calls per sample"="calls per sample (vel)", "index criteria"=w265, "active states"=w264) -> ("encoder position"=w318:i32, "velocity"=w311:i16)  [unwired: 5 in, 2 out]
    n164 = call-poly <vilib>:"nism.incremental.2.vi"("a phase"=w278, "reset"=w269, "b phase"=w277, "z phase"=w276, "calls per sample"="calls per sample (vel)", "index criteria"=w265, "active states"=w264) -> ("encoder position"=w317:i32, "velocity"=w310:i16)  [unwired: 5 in, 2 out]
    n165 = call-poly <vilib>:"nism.incremental.2.vi"("a phase"=w272, "reset"=w269, "b phase"=w271, "z phase"=w270, "calls per sample"="calls per sample (vel)", "index criteria"=w265, "active states"=w264) -> ("encoder position"=w268:i32, "velocity"=w267:i16)  [unwired: 5 in, 2 out]
    n166 = Build Array(w321, w320, w319, w318, w317, w268) -> (w316:i32[])
    n167 = Build Array(w314, w313, w312, w311, w310, w267) -> (w315:i16[])
    n168 = global write "Global FPGA 6-axis.vi" "Unfiltered Position Feedback"(w316) -> ()
    n169 = global write "Global FPGA 6-axis.vi" "Unfiltered Velocity Feedback"(w315) -> ()
  }
  n170 = while "RT Watchdog Loop" {
    shift-right: ["Enable Watchdog"] -> _
    shift-left: FALSE ("Enable RT Watchdog") -> [w336]
    stop <- FALSE stop-if-true
    # "Watchdog Loop"
    n171 = Greater?(x="Enable Watchdog", y=w336) -> (0:w333:bool)
    n172 = case shown="True" "Enable Watchdog" {
      tunnel: w333 -> [_ w339]
      frame False {
        # "This loop has to be explicitly enabled from the RT Main VI.  This reduces the possiblity of an endless reboot cycle."
      }
      frame True {
        # "This boolean is set to \"Latch When Released\""
        # "Compare elapsed time to specified timeout value"
        # "Reset timer when the RT Main VI pets the watchdog or the watchdog is initially enabled"
        n173 = Or(x=w339, y="Pet Watchdog") -> (x .or. y?=w338:bool)
        n174 = call "Tick Count"() -> ("Tick Count(Ticks)"=w342:u32)
        n175 = call "FPGA Watchdog - Elapsed Time.vi"("Reset"=w338, "Timeout Period"="Watchdog Timeout Period (ticks)", "Current Time"=w342) -> ("Timeout"=w337:bool, "Elapsed Time"=→"Time Since Last Pet":u64)  [unwired: 7 in]
        n176 = case shown="True" w337 {
          frame False {
            # "Timeout has not expired."
          }
          frame True {
            # "#CodeRecommended - Ensure that your application behaves safely when System Reset is called. Depending on your chassis, System Reset may not keep the FPGA running or place it in the user-defined safe state. Refer to your chassis documentation to learn how System Reset behaves on your specific hardware."
            # "Timeout has expired. Reset the RT system and put the FPGA into a safe state."
            n177 = local write "Enable Watchdog"(FALSE ("Enable RT Watchdog")) -> ()
            n178 = xnode "FPGA I/O Node"("System Reset"=TRUE ("RT Reset on Watchdog Failure?")) -> ()  [unwired: 1 in, 1 out]
            "Watchdog Timed Out?" <- TRUE ("Watchdog Timed Out?")
          }
        }
      }
    }
  }
  n179 = timed-loop "Synchronization Loop" {
    timing: w7 -> [_]
    timing-out: [_] -> w6
    stop <- FALSE stop-if-true
    n180 = xnode "FPGA I/O Node"() -> ("Scan Clock"=w351:bool)  [unwired: 1 in, 1 out]
    n181 = global read "Global FPGA 6-axis.vi" "Sync Enable"() -> (w350:bool)
    n182 = Select(t="Sync Value", s="Sync Enable override?", f=w350) -> (s? t:f=w347:bool)
    n183 = call-poly <vilib>:"nism.scan.generateSyncScan.vi"("scan enable?"=w347, "scan clock"=w351) -> ("timer control"=w352:T15)  [unwired: 3 in]
    n184 = global write "Global FPGA 6-axis.vi" "Timer Control"(w352) -> ()
  }
  n185 = timed-loop "Reset Monitoring Loop" {
    timing: w5 -> [_]
    timing-out: [_] -> w4
    stop <- FALSE stop-if-true
    n186 = global read "Global FPGA 6-axis.vi" "Reset Pending"() -> (w358:bool[])
    n187 = xnode "FPGA I/O Node"() -> ("Scan Clock"=w357:bool)  [unwired: 1 in, 1 out]
    n188 = feedback-in #1(w357) -> ()
    n189 = feedback #1() -> (w356:bool)  [unwired: 1 in]
    n190 = Greater?(x=w357, y=w356) -> (0:w362:bool)
    n191 = feedback #2() -> (w361:bool[])  [unwired: 1 in]
    n192 = Select(t=w358, s=w362, f=w361) -> (s? t:f=w359:bool[])
    n193 = feedback-in #2(w359) -> ()
    n194 = global write "Global FPGA 6-axis.vi" "Reset"(w359) -> ()
  }
  n195 = node-c288(w4) -> ()
  n196 = node-c288(w6) -> ()
  n197 = node-c288(w1) -> ()
  n198 = disable-structure shown="Disabled" {
    frame Disabled {
      n199 = Index Array() -> (element #1=w369, element #2=w370, element #3=w371, element #4=w372, element #5=w373, element #6=w374)  [unwired: 7 in]
      n200 = Index Array() -> (element #1=w375, element #2=w376, element #3=w377, element #4=w378, element #5=w379, element #6=w380)  [unwired: 7 in]
      n201 = shared-variable "RT Single-Board RIO Target\\User-Defined Variables\\Axis 1.Velocity Feedback"(w369) -> ()  [unwired: 1 in, 1 out]
      n202 = shared-variable "RT Single-Board RIO Target\\User-Defined Variables\\Axis 2.Velocity Feedback"(w370) -> ()  [unwired: 1 in, 1 out]
      n203 = shared-variable "RT Single-Board RIO Target\\User-Defined Variables\\Axis 3.Velocity Feedback"(w371) -> ()  [unwired: 1 in, 1 out]
      n204 = shared-variable "RT Single-Board RIO Target\\User-Defined Variables\\Axis 4.Velocity Feedback"(w372) -> ()  [unwired: 1 in, 1 out]
      n205 = shared-variable "RT Single-Board RIO Target\\User-Defined Variables\\Axis 5.Velocity Feedback"(w373) -> ()  [unwired: 1 in, 1 out]
      n206 = shared-variable "RT Single-Board RIO Target\\User-Defined Variables\\Axis 6.Velocity Feedback"(w374) -> ()  [unwired: 1 in, 1 out]
      n207 = shared-variable "RT Single-Board RIO Target\\User-Defined Variables\\Axis 1.Position Feedback"(w375) -> ()  [unwired: 1 in, 1 out]
      n208 = shared-variable "RT Single-Board RIO Target\\User-Defined Variables\\Axis 2.Position Feedback"(w376) -> ()  [unwired: 1 in, 1 out]
      n209 = shared-variable "RT Single-Board RIO Target\\User-Defined Variables\\Axis 3.Position Feedback"(w377) -> ()  [unwired: 1 in, 1 out]
      n210 = shared-variable "RT Single-Board RIO Target\\User-Defined Variables\\Axis 4.Position Feedback"(w378) -> ()  [unwired: 1 in, 1 out]
      n211 = shared-variable "RT Single-Board RIO Target\\User-Defined Variables\\Axis 5.Position Feedback"(w379) -> ()  [unwired: 1 in, 1 out]
      n212 = shared-variable "RT Single-Board RIO Target\\User-Defined Variables\\Axis 6.Position Feedback"(w380) -> ()  [unwired: 1 in, 1 out]
      n213 = global read "Global FPGA 6-axis.vi" "Unfiltered Velocity Feedback"() -> (w367:i16[])
      n214 = Unbundle By Name("Encoder Config (Manual)") -> ("vel. filter coeffs."=w368:i32[])
      n215 = for {
        tunnel: "Velocity Filter Active?" -> [w384]
        tunnel: w368 -> [w383] mode=indexing
        tunnel: w367 -> [w382] mode=indexing
        tunnel: [w381] -> _ mode=indexing
        n216 = case shown="True" w384 {
          tunnel: w382 -> [w386 w390]
          tunnel: w383 -> [_ _]
          tunnel: [w385 w388] -> w381
          frame False {
            n217 = To Fixed-Point(number=w386) -> (fixed-point=w385:fxp<+/-,64,32>)  [unwired: 1 in]
          }
          frame True {
            n218 = To Fixed-Point(number=w390) -> (fixed-point=w389:fxp<+/-,16,16>)  [unwired: 1 in]
            n219 = xnode "Butterworth Filter"("input data"=w389) -> ("output data"=w387:fxp<+/-,16,16>)  [unwired: 2 in, 1 out]
            n220 = To Fixed-Point(number=w387) -> (fixed-point=w388:fxp<+/-,64,32>)  [unwired: 1 in]
          }
        }
      }
    }
    frame Enabled {
    }
  }
